vi "FPGA_Stepper_Control_Main.vi"() -> ()   [LabVIEW 2019]
uses:
  <vilib>/rvi/Emulation/niFpgaGetClockAttributes.vi
  <vilib>/rvi/Emulation/niFpgaSctlEmulationGetInTimedLoop.vi
  <vilib>/rvi/Emulation/niFpgaEmulationReportErrorSimple.vi
  <vilib>/rvi/eio/common/nirviEmuTemplateMethod_errors.vi
  <vilib>/rvi/Emulation/niFpgaCriticalErrorInLSC.vi
  <vilib>/eio/EIONode/EIONode.xnode
  <vilib>/platform/TimedLoop/XDataNode/XDataNode.xnode
  <vilib>/Platform/TimedLoop/XDataNode/nitl_modes.ctl
  <vilib>/Platform/TimedLoop/XDataNode/XDNodeRunTimeDep.lvlib
  <vilib>/Platform/TimedLoop/XDataNode/wakeup.ctl
  <vilib>/Platform/TimedLoop/XDataNode/timing_clust.ctl
  <vilib>/rvi/FXPMathLib/FxpMul/XNode/nifxpmath_Multiplier.xnode
  <vilib>/rvi/FXPMathLib/sim/FxpSim.dll
panel:
  in  "Stepper Direction":bool
  in  "Stepper Enable":bool
  in  "Half Peirod (pulse 40MHz)":u32 caption="Count(Ticks)"
  in  "stop":bool
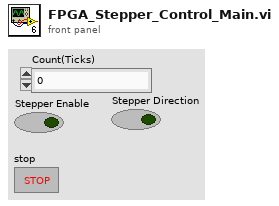
[diagram p1: front panel]
types:
  T1 = typedef "XDNodeRunTimeDep.lvlib/timing_clust.ctl" = cluster{"Expected End [f-1]":u64, "Actual End [f-1]":u64, "Finished Late? [f-1]":bool, "Expected End [i-1]":u64, "Actual End [i-1]":u64, "Finished Late? [i-1]":bool, "Expected Start [i]":u64, "Actual Start [i]":u64, "Expected Start [f]":u64, "Actual Start [f]":u64, "Source Name":string, "Structure Name":string, "Period":i64, "Deadline":i64, "Offset":i64, "Start":i64, "Priority":i32, "Timeout":i32, "Mode":T2, "Wakeup Reason":T3, "Error":errorcluster, "Source Type":string, "Secondary Source Type":string, "Global End Time":u64, "Global Start Time":u64, "Frame Duration":u64, "Iteration Duration":u64, "Assigned CPU":i32, "I/O Scan Engine Mode":u32}
  T2 = typedef "XDNodeRunTimeDep.lvlib/nitl_modes.ctl" = enum32{"No Change", "Process missed periods, maintain original phase", "Discard missed periods, maintain original phase", "Process missed periods, ignore original phase", "Discard missed periods, ignore original phase"}
  T3 = typedef "XDNodeRunTimeDep.lvlib/wakeup.ctl" = enum32{"Normal", "Aborted", "Asynchronous wakeup", "Timing source error", "Timed loop error", "Timeout"}
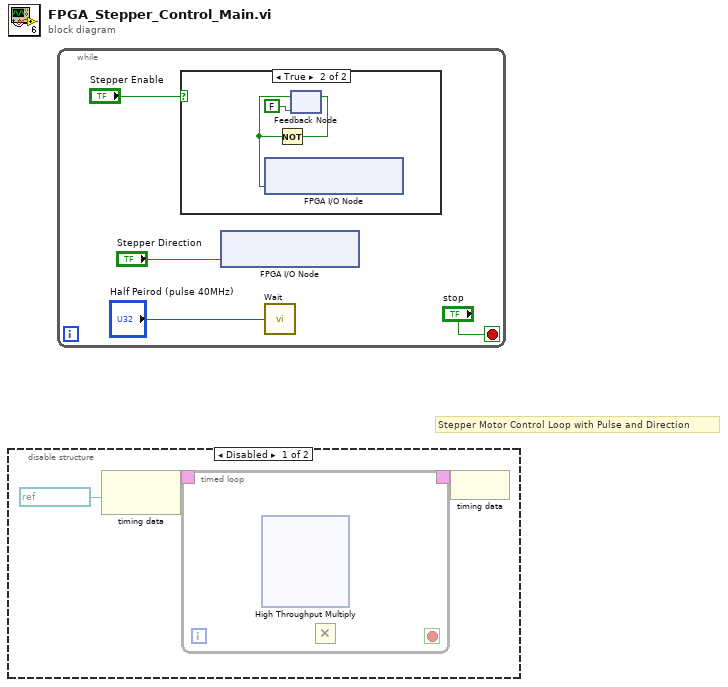
[diagram p0: block diagram]
diagram:
  # "Stepper Motor Control Loop with Pulse and Direction"
  n1 = disable-structure shown="Disabled" {
    frame Disabled {
      n2 = node-c288(refnum<k21> "200MHz" ("Source Name")) -> (w3:T1)
      n3 = timed-loop {
        timing: w3 -> [_]
        timing-out: [_] -> w2
        stop <- _ stop-if-true
        n4 = xnode "High Throughput Multiply"() -> ()  [unwired: 2 in, 1 out]
        n5 = Multiply() -> ()  [unwired: 2 in, 1 out]
      }
      n6 = node-c288(w2) -> ()
    }
    frame Enabled {
    }
  }
  n7 = while {
    stop <- "stop" stop-if-true
    n8 = case shown="True" "Stepper Enable" {
      frame False {
      }
      frame True {
        n9 = feedback #1(FALSE ("Connector0/DIO0")) -> (w14:bool)
        n10 = xnode "FPGA I/O Node"("ConnectorA/DIO0"=w14) -> ()  [unwired: 1 in, 1 out]
        n11 = Not(x=w14) -> (.not. x?=w15:bool)
        n12 = feedback-in #1(w15) -> ()
      }
    }
    n13 = xnode "FPGA I/O Node"("ConnectorA/DIO1"="Stepper Direction") -> ()  [unwired: 1 in, 1 out]
    n14 = call "Wait"("Count(Ticks)"="Half Peirod (pulse 40MHz)") -> ()  [unwired: 1 out]
  }
